vi "UART Config Pane.vi"(6 "_SubPanelMessages":refnum<notifier>, 9 "_myEmbeddedToFrameEvent":T5, 10 "_myEmbedded.Exit":refnum<user-event>, 11 "_Property Bundle":cluster{"Name":string, "Value":variant}[](array[cluster])) -> (1 "_Connection Informations":T1, 2 "_Scripter Input":T7)   [LabVIEW 2021]
doc: "Writes data to or reads data from a Universal Asynchronous Receiver/Transmitter (UART) device."
uses:
  <vilib>/myRIO/Common/Express VI Framework/xctls/myRIO Channel Name/myRIO Channel Name.xctl
  <vilib>/myRIO/Common/Express VI Framework/typedefs/Config Pane to Framework Ref.ctl
  <vilib>/myRIO/Common/Express VI Framework/typedefs/Data Validate Ref.ctl
  <vilib>/myRIO/Common/Express VI Framework/typedefs/Scripter Input.ctl
  <vilib>/myRIO/Common/Express VI Framework/typedefs/WireThrough Terminal Names.ctl
  <vilib>/myRIO/Common/Express VI Framework/typedefs/Instrument Driver Method Descriptor Array.ctl
  <vilib>/myRIO/Common/Express VI Framework/typedefs/Instrument Driver Method Descriptor.ctl
  <vilib>/myRIO/Common/Express VI Framework/typedefs/Sub Panel Messages.ctl
  <vilib>/myRIO/Common/Express VI Framework/typedefs/Connection Informations.ctl
  <vilib>/myRIO/Common/Instrument Driver Framework/Utilities/typedefs/Channel Types.ctl
  <vilib>/myRIO/Instrument Drivers/Onboard IO/UART/typedef/VISA Configuration.ctl
  <vilib>/myRIO/Instrument Drivers/Onboard IO/UART/UART.lvlib
panel:
  in  "Read all Available?":bool
  in  "Mode":enum32{"Write", "Read"}(radio) caption="Mode:"
  in  "Baud rate:":u32(ring)=9600 items=["110"=110, "300"=300, "600"=600, "1,200"=1200, "2,400"=2400, "4,800"=4800, "9,600"=9600, "19,200"=19200, "38,400"=38400, "57,600"=57600, "115,200"=115200, "230,400"=230400]
  in  "Stop bits:":u16(ring)=10 items=["1.0"=10, "2.0"=20]
  in  "Parity:":u16(ring) items=["Even"=2, "Odd"=1, "None"=0]
  in  "Data bits:":u16(ring)=8 items=["7"=7, "8"=8]
  out "_Channel Details:":string caption="Connections:"
  in  "Channel:":u16(xcontrol)
  in  "_Default Alias String":string
  in  "_VI Default Name (Edit and make value default)":string="UART"
  in  "Name:":string caption="Node name:"
  in  "_WireThrough Info (Edit and make value default)":T2={"WireThrough Top In"="VISA resource name in", "WireThrough Bottom In"="error in (no error)", "WireThrough Top Out"="VISA resource name out", "WireThrough Bottom Out"="error out"}
  in  "_Template Array (Edit and make value default)":T3=[{"Function Name"="Open", "VI Path"=path "<vilib>/myRIO/Instrument Drivers/Onboard IO/UART/vis", "Script"=FALSE, "Inputs"=[{"name"="VISA resource name in", "value"=variant, "Config Pane Only"=TRUE, "Build Array"=FALSE, "Bundle Cluster"=FALSE, "Show Term"=FALSE, "alias"=[], "Required Input"=FALSE}], "Outputs"=[], "VI Class"=enum."Open", "Controls Refs[]"=[], "Inline"=FALSE}, {"Function Name"="Configure", "VI Path"=path "<vilib>/myRIO/Instrument Drivers/Onboard IO/UART/vis", "Script"=TRUE, "Inputs"=[{"name"="VISA resource name in", "value"=variant, "Config Pane Only"=TRUE, "Build Array"=FALSE, "Bundle Cluster"=FALSE, "Show Term"=FALSE, "alias"=[], "Required Input"=FALSE}, {"name"="VISA Configuration", "value"=variant, "Config Pane Only"=TRUE, "Build Array"=FALSE, "Bundle Cluster"=FALSE, "Show Term"=FALSE, "alias"=[], "Required Input"=FALSE}], "Outputs"=[], "VI Class"=enum."Configure", "Controls Refs[]"=[], "Inline"=TRUE}, {"Function Name"="Write", "VI Path"=path "<vilib>/myRIO/Instrument Drivers/Onboard IO/UART/vis", "Script"=FALSE, "Inputs"=[{"name"="Characters to Write", "value"=variant, "Config Pane Only"=FALSE, "Build Array"=FALSE, "Bundle Cluster"=FALSE, "Show Term"=TRUE, "alias"=[], "Required Input"=TRUE}], "Outputs"=[{"name"="Character Count", "value"=variant, "Show Term"=TRUE, "Index Array"=FALSE, "Unbundle Cluster"=FALSE, "alias"=[]}], "VI Class"=enum."Data", "Controls Refs[]"=[], "Inline"=TRUE}, {"Function Name"="Read", "VI Path"=path "<vilib>/myRIO/Instrument Drivers/Onboard IO/UART/vis", "Script"=FALSE, "Inputs"=[{"name"="Character Count", "value"=variant, "Config Pane Only"=FALSE, "Build Array"=FALSE, "Bundle Cluster"=FALSE, "Show Term"=TRUE, "alias"=[], "Required Input"=FALSE}], "Outputs"=[{"name"="Characters Read", "value"=variant, "Show Term"=TRUE, "Index Array"=FALSE, "Unbundle Cluster"=FALSE, "alias"=[]}], "VI Class"=enum."Data", "Controls Refs[]"=[], "Inline"=TRUE}, {"Function Name"="Read All", "VI Path"=path "<vilib>/myRIO/Instrument Drivers/Onboard IO/UART/vis", "Script"=FALSE, "Inputs"=[], "Outputs"=[{"name"="Characters Read", "value"=variant, "Show Term"=TRUE, "Index Array"=FALSE, "Unbundle Cluster"=FALSE, "alias"=[]}], "VI Class"=enum."Data", "Controls Refs[]"=[], "Inline"=TRUE}, {"Function Name"="Close", "VI Path"=path "<vilib>/myRIO/Instrument Drivers/Onboard IO/UART/vis", "Script"=FALSE, "Inputs"=[], "Outputs"=[], "VI Class"=enum."Close", "Controls Refs[]"=[], "Inline"=TRUE}, {"Function Name"="Close UART", "VI Path"=path "<vilib>/myRIO/Instrument Drivers/Onboard IO/UART/vis", "Script"=FALSE, "Inputs"=[], "Outputs"=[], "VI Class"=enum."Close", "Controls Refs[]"=[], "Inline"=TRUE}]
  in  "_Test Close":bool
  # "User Visible Area"
  # "NOTE: Tab Order has been set\nfor this Front Panel.\n\nSee Edit>>Set Tabbing Order...\n\nAll controls that are not visible at \nruntime are excluded from Tabbing order\n\nTo exlude a control from context\nhelp prefix its label text with a '-'"
  # "Communication settings"
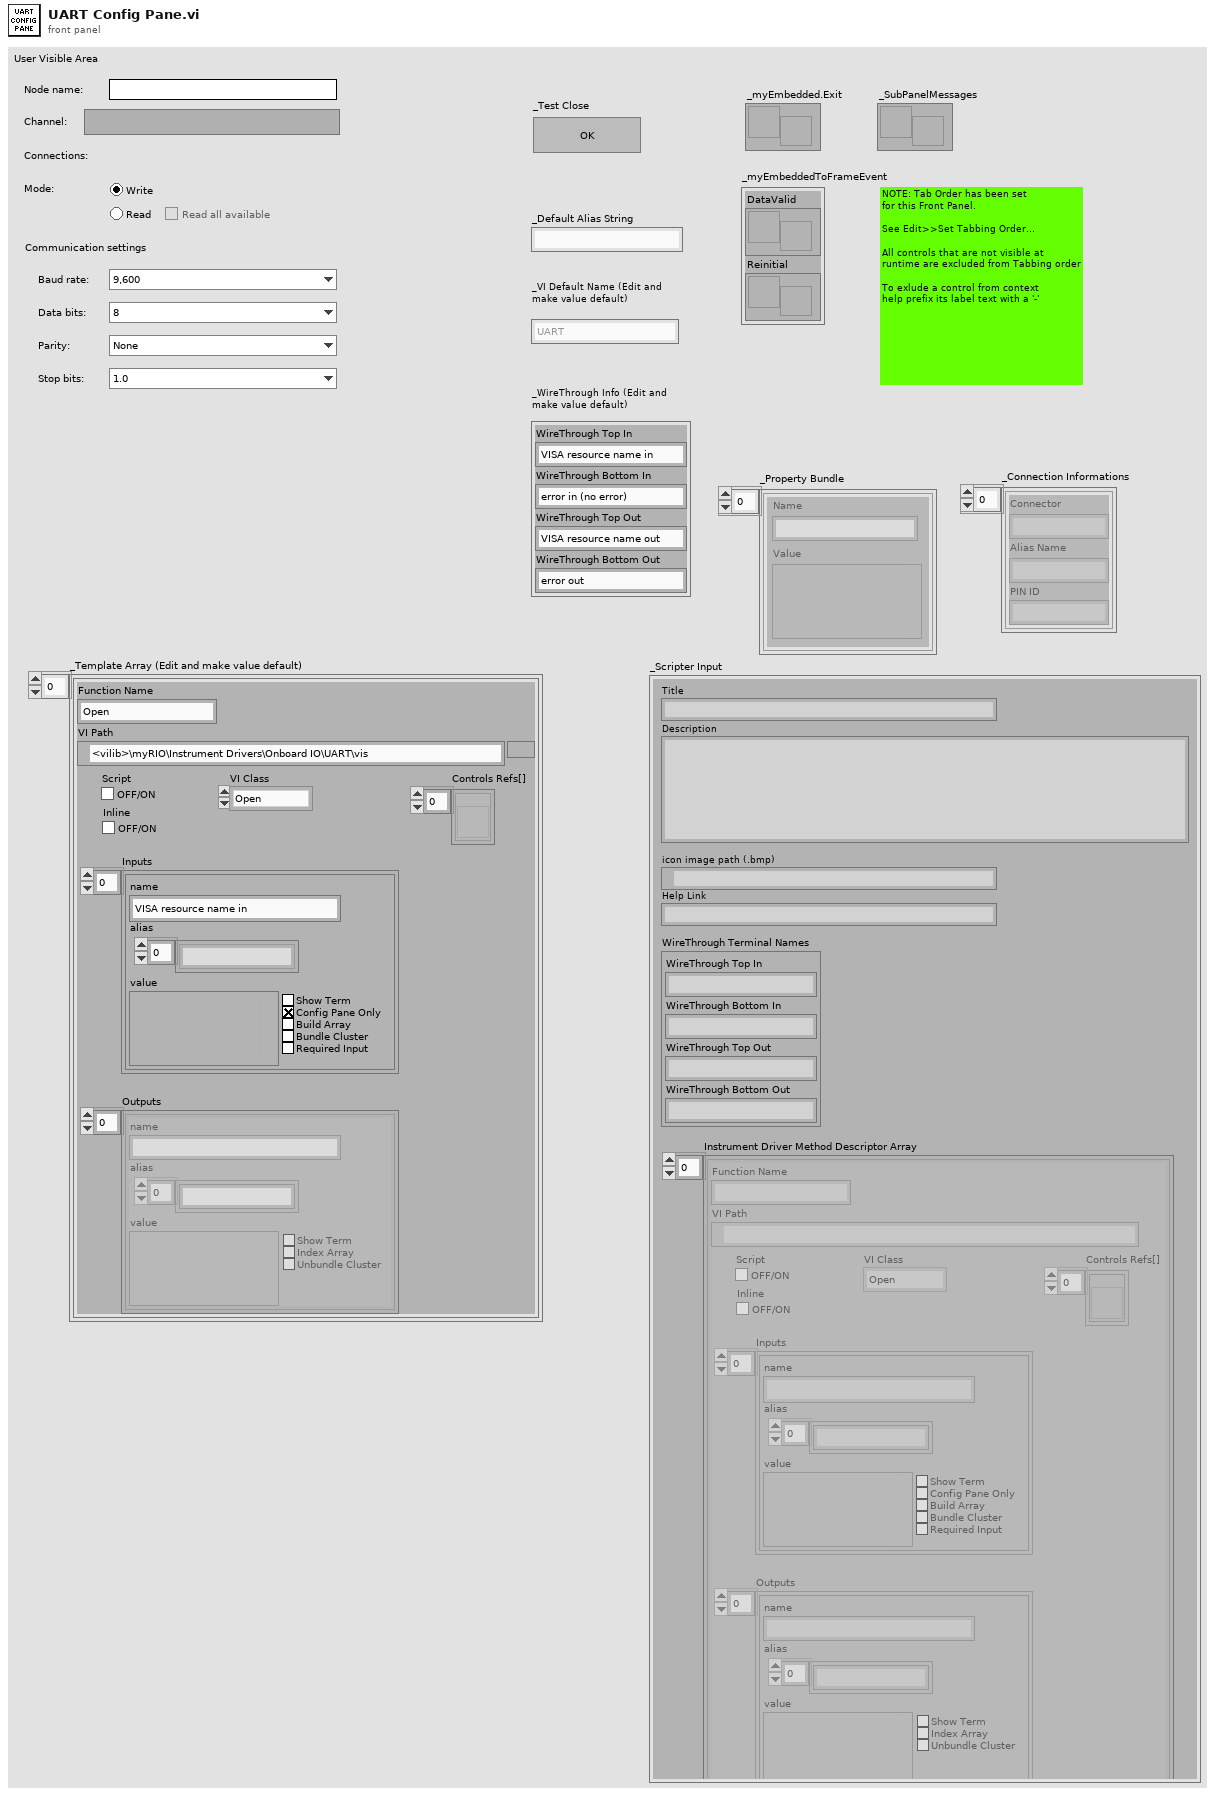
[diagram p1: front panel]
types:
  T1 = typedef "Connection Informations.ctl" = cluster{"Connector":string, "Alias Name":string, "PIN ID":string}[]
  T2 = typedef "WireThrough Terminal Names.ctl" = cluster{"WireThrough Top In":string, "WireThrough Bottom In":string, "WireThrough Top Out":string, "WireThrough Bottom Out":string}
  T3 = typedef "Instrument Driver Method Descriptor Array.ctl" = T4[]
  T4 = typedef "Instrument Driver Method Descriptor.ctl" = cluster{"Function Name":string, "VI Path":path, "Script":bool, "Inputs":cluster{"name":string, "value":variant, "Config Pane Only":bool, "Build Array":bool, "Bundle Cluster":bool, "Show Term":bool, "alias":string[], "Required Input":bool}[], "Outputs":cluster{"name":string, "value":variant, "Show Term":bool, "Index Array":bool, "Unbundle Cluster":bool, "alias":string[]}[], "VI Class":enum16{"Open", "Configure", "Data", "Manage", "Close"}, "Controls Refs[]":refnum<vi>[], "Inline":bool}
  T5 = typedef "Config Pane to Framework Ref.ctl" = cluster{"DataValid":T6, "Reinitial":refnum<user-event>}
  T6 = typedef "Data Validate Ref.ctl" = refnum<user-event>
  T7 = typedef "Scripter Input.ctl" = cluster{"Title":string, "Description":string, "icon image path (.bmp)":path, "Help Link":string, "WireThrough Terminal Names":T2, "Instrument Driver Method Descriptor Array":T3}
  T8 = enum8{"Enabled", "Disabled", "Disabled and Grayed Out"}
  T9 = typedef "Channel Types.ctl" = enum32{"Unknown", "AI", "AO", "DIO - DI", "DIO", "DIO - DO", "I2C", "PWM", "Encoder", "SPI", "UART", "Accelerometer", "DIO - LED", "DIO - Button", "AI (N Samples)", "AudioIn (N Samples)", "AO (N Samples)", "AudioOut (N Samples)", "DI (N Samples)", "DO (N Samples)", "AI IRQ", "DI IRQ", "Timer IRQ", "RSL", "Relay", "CAN", "AI (Continuous)", "AO (Continuous)"}
  T10 = typedef "Channel Info.ctl" = cluster{"Channel Name":string, "Alias":string, "Used?":bool, "Not Support?":bool, "Property Bundle":cluster{"Name":string, "Value":variant}[]}
  T11 = typedef "LVStringsAndValuesArrayTypeDef_U32.ctl" = cluster{"String":string, "Value":u32}[]
  T12 = typedef "Sub Panel Messages.ctl" = enum16{"Initialized"}
  T13 = cluster{"Connector":string, "Alias Name":string, "PIN ID":string}
  T14 = typedef "UART.lvlib/VISA Configuration.ctl" = cluster{"baud rate (9600)":u32, "data bits (8)":u16, "parity (0:none)":enum16{"None", "Odd", "Even", "Mark", "Space"}, "stop bits (10: 1 bit)":u16, "flow control (0:none)":u16, "termination char\n(0xA = '\\n' = LF) ":u8, "Enable Termination\nChar (T)":bool, "timeout (10sec)":u32}
  T15 = cluster{"name":string, "value":variant, "Config Pane Only":bool, "Build Array":bool, "Bundle Cluster":bool, "Show Term":bool, "alias":string[], "Required Input":bool}[]
  T16 = cluster{"name":string, "value":variant, "Config Pane Only":bool, "Build Array":bool, "Bundle Cluster":bool, "Show Term":bool, "alias":string[], "Required Input":bool}
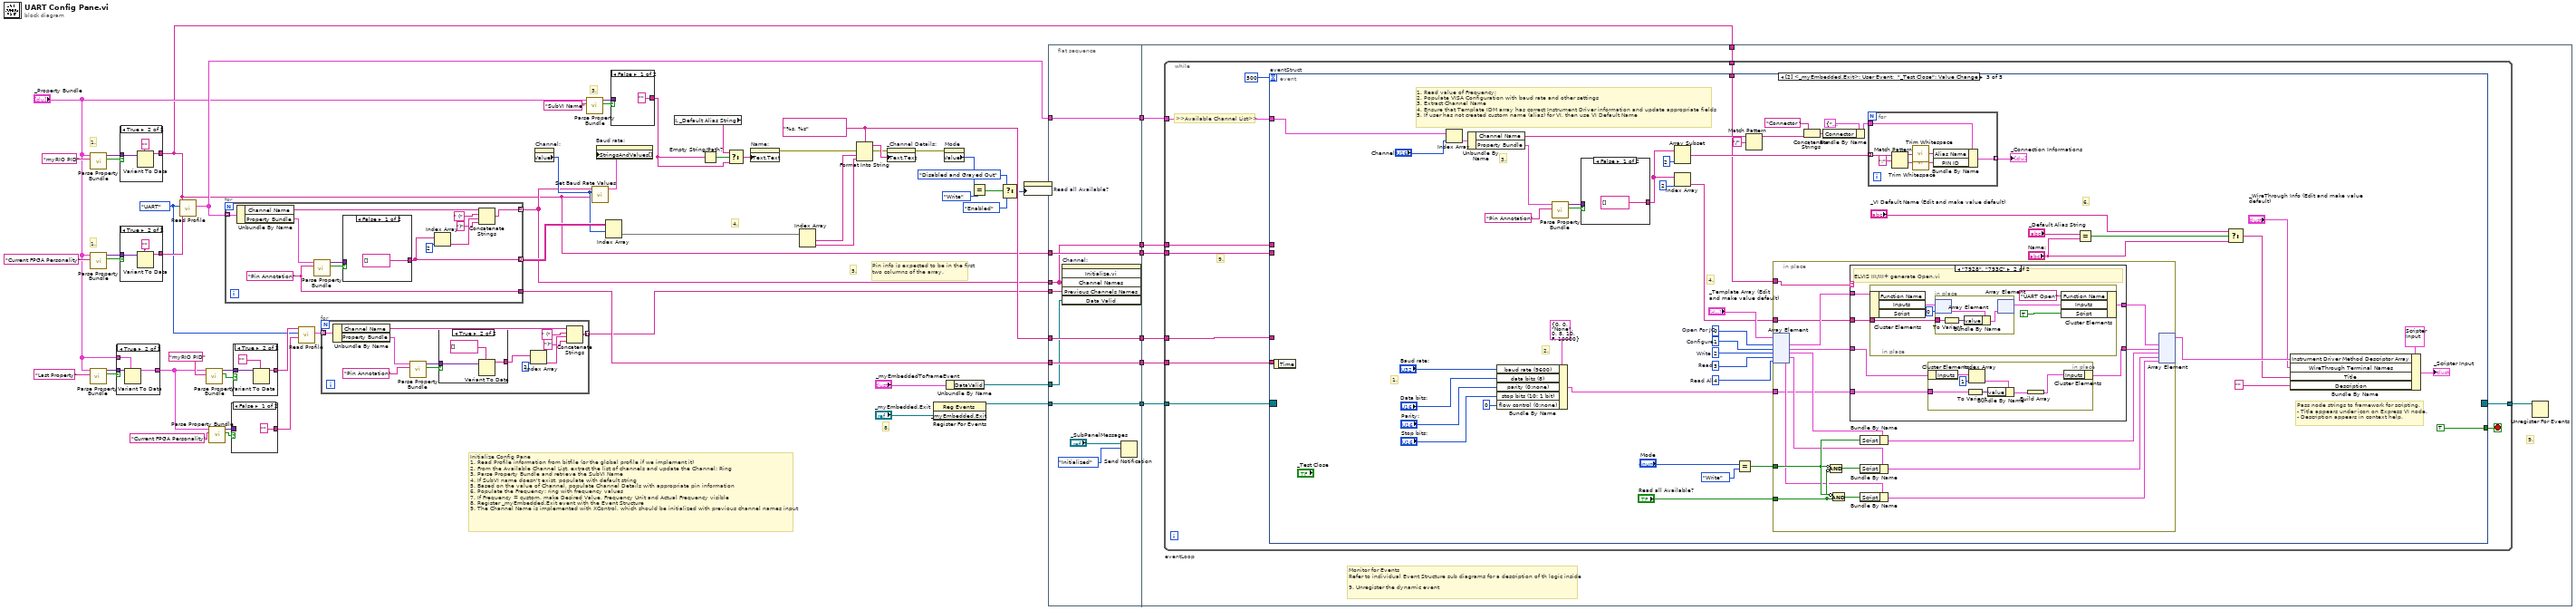
[diagram p0: block diagram]
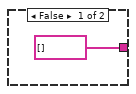
[diagram p2: hidden frame]
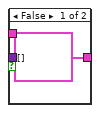
[diagram p3: hidden frame]
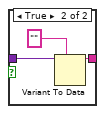
[diagram p4: hidden frame]
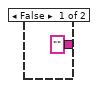
[diagram p5: hidden frame]
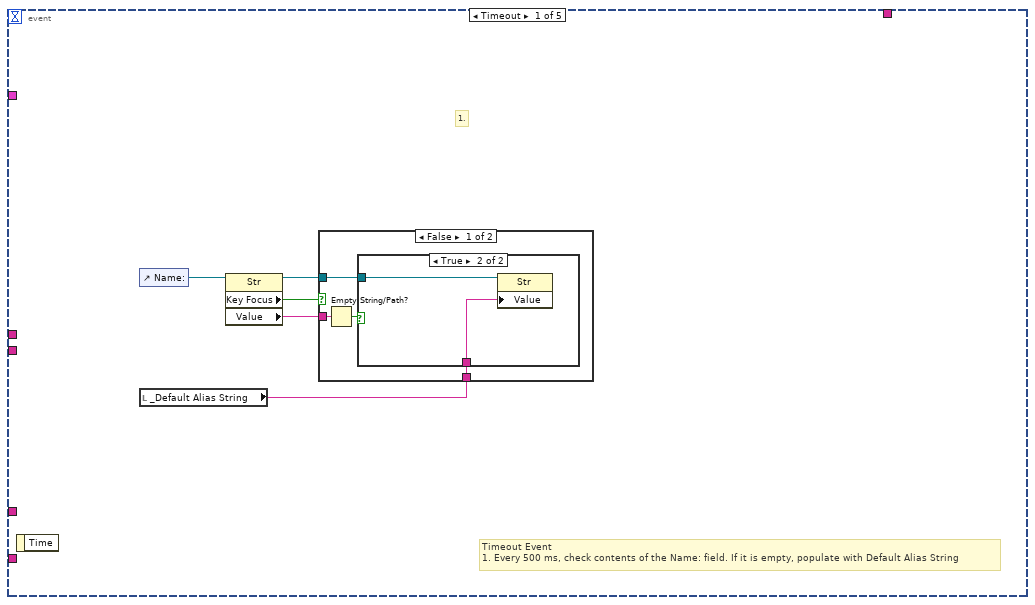
[diagram p6: hidden frame]
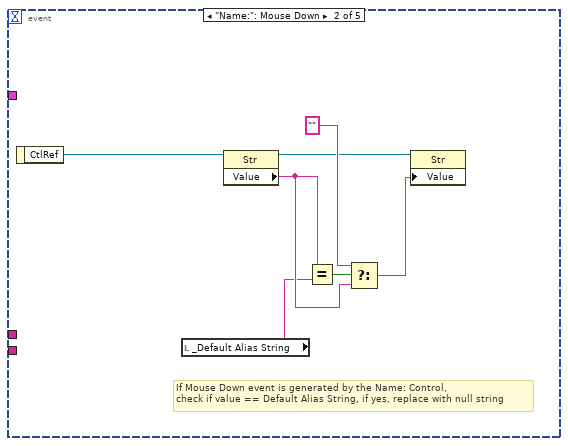
[diagram p9: hidden frame]
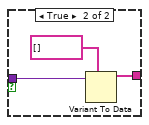
[diagram p10: hidden frame]
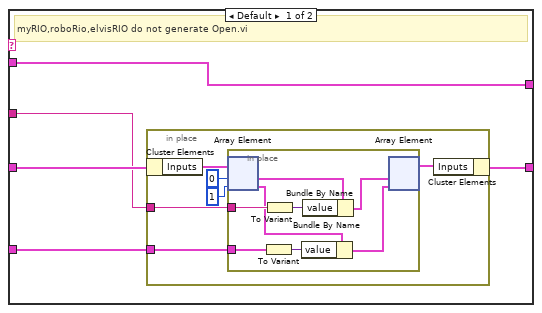
[diagram p11: hidden frame]
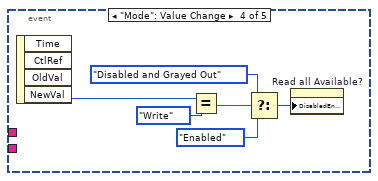
[diagram p12: hidden frame]
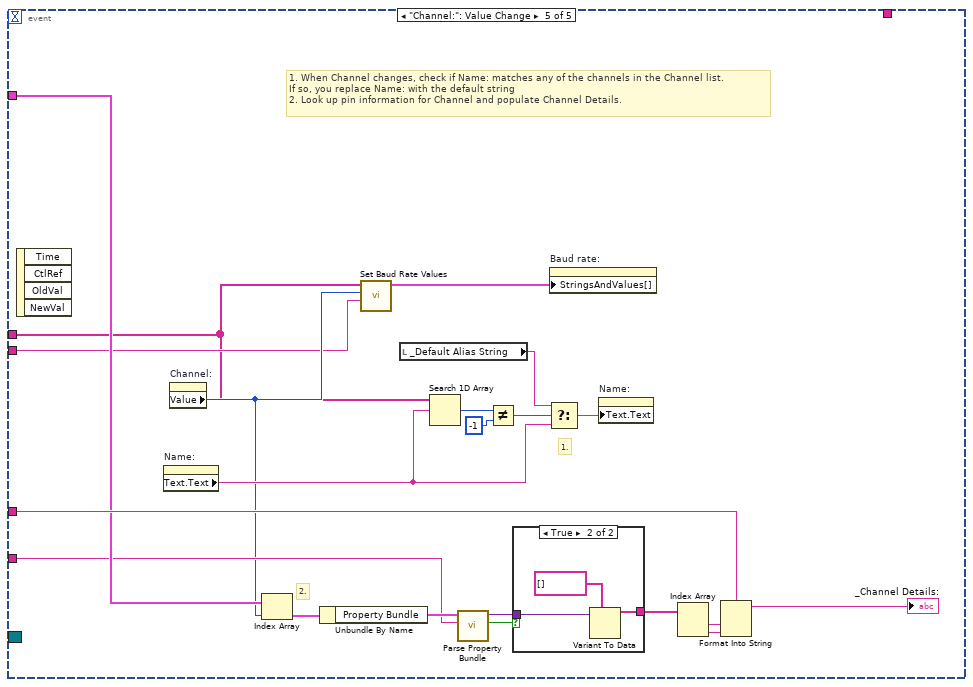
[diagram p13: hidden frame]
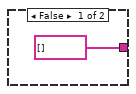
[diagram p14: hidden frame]
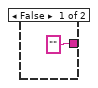
[diagram p15: hidden frame]
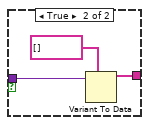
[diagram p16: hidden frame]
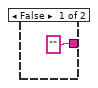
[diagram p17: hidden frame]
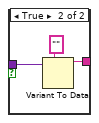
[diagram p18: hidden frame]
diagram:
  w9 = Channel_Types."UART" ("Channel to Read")
  w50 = "%s, %s"
  # "1."
  # "Pin info is expected to be in the first two columns of the array."
  # "1."
  # "8."
  # "5."
  # "4."
  # "3."
  # "Initialize Config Pane\n1. Read Profile information from bitfile (or the global profile if we implement it)\n2. From the Available Channel List, extract the list of channels and update the Channel: Ring\n3. Parse Property Bundle and retrieve the SubVI Name\n4. If SubVI name doesn't exist, populate with default string\n5. Based on the value of Channel, populate Channel Details with appropriate pin information\n6. Populate the Frequency: ring with frequency values\n7. If Frequency = custom, make Desired Value, Frequency Unit and Actual Frequency visible\n8. Register _myEmbedded.Exit event with the Event Structure \n9. The Channel Name is implemented with XControl, which should be initialized with previous channel names input"
  n1 = call <vilib>:"Parse Property Bundle.vi"("Name"="Last Property", "Property Bundle"="_Property Bundle") -> ("Found?"=w12:bool, "Value"=w13:variant)  [unwired: 8 in]
  n2 = call <vilib>:"Parse Property Bundle.vi"("Name"="myRIO PID", "Property Bundle"="_Property Bundle") -> ("Found?"=w45:bool, "Value"=w46:variant)  [unwired: 8 in]
  n3 = call <vilib>:"Parse Property Bundle.vi"("Name"="Current FPGA Personality", "Property Bundle"="_Property Bundle") -> ("Found?"=w32:bool, "Value"=w31:variant)  [unwired: 8 in]
  n4 = case shown="True" w12 {
    tunnel: w13 -> [_ w65]
    tunnel: [cluster{"Name":string, "Value":variant}[] [] ("_Property Bundle") w64] -> w11
    tunnel: "_Property Bundle" -> [_ w63]
    frame False {
    }
    frame True {
      n5 = Variant To Data(type=w63, Variant=w65) -> (data=w64:cluster{"Name":string, "Value":variant}[])  [unwired: 1 in, 1 out]
    }
  }
  n6 = case shown="True" w45 {
    tunnel: w46 -> [_ w69]
    tunnel: ["" ("Name") w67] -> w1
    frame False {
    }
    frame True {
      n7 = Variant To Data(type="" ("Name"), Variant=w69) -> (data=w67:string)  [unwired: 1 in, 1 out]
    }
  }
  n8 = case shown="True" w32 {
    tunnel: w31 -> [_ w73]
    tunnel: ["" ("Name") w71] -> w29
    frame False {
    }
    frame True {
      n9 = Variant To Data(type="" ("Name"), Variant=w73) -> (data=w71:string)  [unwired: 1 in, 1 out]
    }
  }
  n10 = call <vilib>:"Read Profile.vi"("FPGA Name"=w29, "Channel to Read"=w9, "myRIO PID"=w1) -> ("Channel List Out"=w44:T10[])  [unwired: 7 in, 1 out]
  n11 = call <vilib>:"Parse Property Bundle.vi"("Name"="myRIO PID", "Property Bundle"=w11) -> ("Found?"=w21:bool, "Value"=w20:variant)  [unwired: 8 in]
  n12 = call <vilib>:"Parse Property Bundle.vi"("Name"="Current FPGA Personality", "Property Bundle"=w11) -> ("Found?"=w16:bool, "Value"=w17:variant)  [unwired: 8 in]
  n13 = for {
    tunnel: [w83] -> w3 mode=indexing
    tunnel: w44 -> [w85] mode=indexing
    tunnel: [w79] -> w41 mode=indexing
    tunnel: [w80] -> w42
    w80 = "Pin Annotation" ("Name")
    n14 = Unbundle By Name(w85) -> ("Channel Name"=w84:string, "Property Bundle"=w77:cluster{"Name":string, "Value":variant}[])
    n15 = call <vilib>:"Parse Property Bundle.vi"("Name"=w80, "Property Bundle"=w77) -> ("Found?"=w81:bool, "Value"=w82:variant)  [unwired: 8 in]
    n16 = case shown="False" w81 {
      tunnel: w82 -> [_ w89]
      tunnel: [string[] [] w88] -> w79
      frame False {
      }
      frame True {
        n17 = Variant To Data(type=string[] [], Variant=w89) -> (data=w88:string[])  [unwired: 1 in, 1 out]
      }
    }
    n18 = Index Array(array=w79, index=2) -> (element=w76:string)
    n19 = Concatenate Strings(w84, " (" ("string"), w76, ")" ("string")) -> (w83:string)
  }
  n20 = case shown="False" w16 {
    tunnel: w17 -> [_ w93]
    tunnel: ["" ("Name") w91] -> w15
    frame False {
    }
    frame True {
      n21 = Variant To Data(type="" ("Name"), Variant=w93) -> (data=w91:string)  [unwired: 1 in, 1 out]
    }
  }
  n22 = case shown="True" w21 {
    tunnel: w20 -> [_ w97]
    tunnel: ["" ("Name") w95] -> w22
    frame False {
    }
    frame True {
      n23 = Variant To Data(type="" ("Name"), Variant=w97) -> (data=w95:string)  [unwired: 1 in, 1 out]
    }
  }
  n24 = call <vilib>:"Read Profile.vi"("FPGA Name"=w15, "Channel to Read"=w9, "myRIO PID"=w22) -> ("Channel List Out"=w8:T10[])  [unwired: 7 in, 1 out]
  n25 = for {
    tunnel: [w107] -> w2 mode=indexing
    tunnel: w8 -> [w109] mode=indexing
    n26 = Unbundle By Name(w109) -> ("Channel Name"=w108:string, "Property Bundle"=w101:cluster{"Name":string, "Value":variant}[])
    n27 = call <vilib>:"Parse Property Bundle.vi"("Name"="Pin Annotation", "Property Bundle"=w101) -> ("Found?"=w105:bool, "Value"=w106:variant)  [unwired: 8 in]
    n28 = case shown="True" w105 {
      tunnel: w106 -> [_ w113]
      tunnel: [string[] [] w112] -> w103
      frame False {
      }
      frame True {
        n29 = Variant To Data(type=string[] [], Variant=w113) -> (data=w112:string[])  [unwired: 1 in, 1 out]
      }
    }
    n30 = Index Array(array=w103, index=2) -> (element=w100:string)
    n31 = Concatenate Strings(w108, " (" ("string"), w100, ")" ("string")) -> (w107:string)
  }
  n32 = property on="Channel:" class="myRIO Channel Name (strict)"() -> ("Value"=w4:u16)  [unwired: 2 in, 2 out]
  n33 = call <vilib>:"Parse Property Bundle.vi"("Name"="SubVI Name", "Property Bundle"="_Property Bundle") -> ("Found?"=w56:bool, "Value"=w55:variant)  [unwired: 8 in]
  n34 = call <vilib>:"Set Baud Rate Values.vi"("PID"=w1, "Channel Index"=w4, "Channel Str"=w3) -> ("Baud Rate Strings And Values"=w24:T11)  [unwired: 8 in]
  n35 = property on="Baud rate:" class="Ring (strict)"("StringsAndValues[]"=w24) -> ()  [unwired: 2 in, 2 out]
  n36 = Index Array(array=w41, index (row)=w4) -> (element=w40:string[])  [unwired: 1 in]
  n37 = case shown="False" w56 {
    tunnel: w55 -> [_ w117]
    tunnel: ["" ("Name") w115] -> w54
    frame False {
    }
    frame True {
      n38 = Variant To Data(type="" ("Name"), Variant=w117) -> (data=w115:string)  [unwired: 1 in, 1 out]
    }
  }
  n39 = local read "_Default Alias String"() -> (w58:string)
  n40 = Empty String/Path?(string/path=w54) -> (empty?=w59:bool)
  n41 = Select(t=w58, s=w59, f=w54) -> (s? t:f=w43:string)
  n42 = property on="Name:" class="Str"("Text.Text"=w43) -> (error out=w53:errorcluster)  [unwired: 2 in, 1 out]
  n43 = Index Array(array=w40) -> (element #1=w49:string, element #2=w48:string)  [unwired: 2 in]
  n44 = Format Into String(format string=w50, error in=w53, w49, w48) -> (resulting string=w52:string, error out=w51:errorcluster)  [unwired: 1 in]
  n45 = property on="_Channel Details:" class="Str"(error in=w51, "Text.Text"=w52) -> (error out=w34:errorcluster)  [unwired: 1 in, 1 out]
  n46 = register-events("_myEmbedded.Exit") -> (reference out=w61:refnum<event-registration>)  [unwired: 2 in, 1 out]
  n47 = property on="Mode" class="RadioBtnsControl (strict)"(error in=w34) -> ("Value"=w33:enum32{"Write", "Read"})  [unwired: 1 in, 2 out]
  n48 = Unbundle By Name("_myEmbeddedToFrameEvent") -> ("DataValid"=w6:T6)
  n49 = Equal?(x=w33, y=enum32{"Write", "Read"}."Write") -> (x = y?=w36:bool)
  n50 = Select(t=T8."Disabled and Grayed Out", s=w36, f=T8."Enabled" ("Disabled")) -> (s? t:f=w39:T8)
  n51 = property on="Read all Available?" class="Bool (strict)"("DisabledEnum"=w39) -> ()  [unwired: 2 in, 2 out]
  n52 = flat-sequence {
    tunnel: w42 -> [w124]
    tunnel: w44 -> [w125]
    tunnel: w50 -> [w126]
    tunnel: w61 -> [w127]
    tunnel: [w127] -> w28
    tunnel: [w126] -> w27
    tunnel: [w125] -> w26
    tunnel: [w124] -> w25
    tunnel: [w121] -> w23
    tunnel: w1 -> [w121]
    tunnel: w6 -> [w118]
    tunnel: w2 -> [w119]
    tunnel: w3 -> [w120]
    tunnel: [w120] -> w5
    tunnel: w28 -> [w135]
    tunnel: w27 -> [w133]
    tunnel: w26 -> [w132]
    tunnel: w25 -> [w131]
    tunnel: w23 -> [w130]
    tunnel: w5 -> [w129]
    tunnel: w1 -> [w128]
    frame #0 {
      n53 = invoke on="Channel:" class="myRIO Channel Name (strict)" method="Initialize.vi"("Channel Names"=w120, "Previous Channels Names"=w119, "Data Valid"=w118) -> ()  [unwired: 3 in, 6 out]
      n54 = Send Notification(notification=Sub_Panel_Messages."Initialized", notifier="_SubPanelMessages") -> ()  [unwired: 1 in, 2 out]
    }
    frame #1 {
      # "9."
      # "Monitor for Events\nRefer to individual Event Structure sub diagrams for a description of th logic inside\n\n9. Unregister the dynamic event"
      n55 = while "eventLoop" {
        tunnel: w135 -> [w144]
        tunnel: [w143] -> w134
        tunnel: w132 -> [w141]
        tunnel: w133 -> [w140]
        tunnel: w131 -> [w139]
        tunnel: w130 -> [w138]
        tunnel: w129 -> [w137]
        tunnel: w128 -> [w136]
        stop <- w145 stop-if-true
        # "9."
        # ">>Available Channel List>>"
        n56 = event "eventStruct" shown="[2] <_myEmbedded.Exit>: User Event;  \"_Test Close\": Value Change" {
          selector: w144 -> [_ _ _ _ _]
          dyn-events: [_ _ _ _ _] -> w143
          timeout: 500 -> [_ _ _ _ _]
          tunnel: [_ _ TRUE ("_Test Close") _ _] -> w145
          tunnel: w141 -> [_ _ w211 _ w296]
          tunnel: w140 -> [_ _ _ _ w303]
          tunnel: w139 -> [_ _ _ _ w295]
          tunnel: w138 -> [_ _ _ _ w291]
          tunnel: w137 -> [_ _ _ _ w290]
          tunnel: w136 -> [_ _ w166 _ _]
          event Timeout {
            # "Timeout Event\n1. Every 500 ms, check contents of the Name: field. If it is empty, populate with Default Alias String"
            # "1."
            n57 = event-data() -> ()  [unwired: 1 in, 1 out]
            n58 = control-ref of="Name:"() -> (w148:refnum<vi>)
            n59 = local read "_Default Alias String"() -> (w146:string)
            n60 = property on="Property Node" class="Str"(reference=w148) -> (reference out=w147:refnum<vi>, "Key Focus"=w149:bool, "Value"=w150:string)  [unwired: 1 in, 1 out]
            n61 = case shown="False" w149 {
              tunnel: w150 -> [w154 _]
              tunnel: w147 -> [w152 _]
              tunnel: w146 -> [w151 _]
              frame False {
                n62 = Empty String/Path?(string/path=w154) -> (empty?=w153:bool)
                n63 = case shown="True" w153 {
                  tunnel: w152 -> [_ w156]
                  tunnel: w151 -> [_ w155]
                  frame False {
                  }
                  frame True {
                    n64 = property on="Property Node" class="Str"(reference=w156, "Value"=w155) -> ()  [unwired: 1 in, 2 out]
                  }
                }
              }
              frame True {
              }
            }
          }
          event "Name:": Mouse Down {
            # "If Mouse Down event is generated by the Name: Control,\ncheck if value == Default Alias String, if yes, replace with null string"
            n65 = event-data() -> ("CtlRef"=w163:refnum<vi>)  [unwired: 1 in]
            n66 = local read "_Default Alias String"() -> (w157:string)
            n67 = property class="Str"(reference=w163) -> (reference out=w159:refnum<vi>, "Value"=w158:string)  [unwired: 1 in, 1 out]
            n68 = Equal?(x=w158, y=w157) -> (x = y?=w162:bool)
            n69 = Select(t="", s=w162, f=w158) -> (s? t:f=w160:string)
            n70 = property class="Str"(reference=w159, "Value"=w160) -> ()  [unwired: 1 in, 2 out]
          }
          event User Event; "_Test Close": Value Change {
            w167 = 0  # Open For JC
            w179 = 4  # Read All
            w190 = 3  # Read
            w210 = 2  # Write
            w207 = 1  # Configure
            # "3."
            # "2."
            # "1. Read value of Frequency:\n2. Populate VISA Configuration with baud rate and other settings\n3. Extract Channel Name\n4. Ensure that Template IDM array has correct Instrument Driver information and update appropriate fields\n5. If user has not created custom name (alias) for VI, then use VI Default Name"
            # "6."
            # "4."
            # "1."
            # "Pass node strings to framework for scripting.\n- Title appears under icon on Express VI node.\n- Description appears in context help."
            n71 = event-data() -> ()  [unwired: 1 in, 1 out]
            n72 = Index Array(array=w211, index="Channel:") -> (element=w188:T10)
            n73 = Unbundle By Name(w188) -> ("Channel Name"=w169:string, "Property Bundle"=w183:cluster{"Name":string, "Value":variant}[])
            n74 = Bundle By Name(cluster=T14 {"baud rate (9600)"=0, "data bits (8)"=0, "parity (0:none)"=enum."None", "stop bits (10: 1 bit)"=0, "flow control (0:none)"=8, "termination char\n(0xA = '\\n' = LF) "=10, "Enable Termination\nChar (T)"=FALSE, "timeout (10sec)"=10000} ("VISA Configuration"), "baud rate (9600)"="Baud rate:", "data bits (8)"="Data bits:", "parity (0:none)"="Parity:", "stop bits (10: 1 bit)"="Stop bits:", "flow control (0:none)"=u16 0) -> (w164:T14)
            n75 = call <vilib>:"Parse Property Bundle.vi"("Name"="Pin Annotation", "Property Bundle"=w183) -> ("Found?"=w186:bool, "Value"=w187:variant)  [unwired: 8 in]
            n76 = case shown="False" w186 {
              tunnel: w187 -> [_ w224]
              tunnel: [string[] [] w223] -> w172
              frame False {
              }
              frame True {
                n77 = Variant To Data(type=string[] [], Variant=w224) -> (data=w223:string[])  [unwired: 1 in, 1 out]
              }
            }
            n78 = Array Subset(array=w172, length=2) -> (w170:string[])  [unwired: 1 in]
            n79 = Index Array(array=w172, index=2) -> (element=w165:string)
            n80 = Equal?(x="Mode", y=enum32{"Write", "Read"}."Write") -> (x = y?=w181:bool)
            n81 = Match Pattern(string=w169, regular expression="/") -> (before substring=w176:string)  [unwired: 1 in, 3 out]
            n82 = in-place {
              in-place-border: w181 -> [w241]
              in-place-border: "Read all Available?" -> [w236]
              in-place-border: w166 -> [w231]
              in-place-border: w165 -> [w227]
              in-place-border: w164 -> [w226]
              n83 = in-place-array #1("_Template Array (Edit and make value default)", w167, w207, w210, w190, w179) -> (w230:T4, w225:T4, w240:T4, w239:T4, w235:T4)
              n84 = Compound Arithmetic op=AND(invert w241, invert w236) -> (w233:bool)
              n85 = Compound Arithmetic op=AND(invert w241, w236) -> (w232:bool)
              n86 = case shown="\"7928\", \"793C\"" w231 {
                tunnel: w230 -> [w246 w265]
                tunnel: [w246 w263] -> w229
                tunnel: [w243 w266] -> w228
                tunnel: w227 -> [w242 w264]
                tunnel: w226 -> [w245 w261]
                tunnel: w225 -> [w244 w262]
                frame Default {
                  # "myRIO,roboRio,elvisRIO do not generate Open.vi"
                  n87 = in-place {
                    in-place-border: w242 -> [w251]
                    in-place-border: w245 -> [w247]
                    n88 = in-place-cluster #2(w244) -> ("Inputs"=w252:T15)
                    n89 = in-place {
                      in-place-border: w251 -> [w257]
                      in-place-border: w247 -> [w253]
                      n90 = in-place-array #3(w252, 0, 1) -> (w260:T16, w255:T16)
                      n91 = To Variant(anything=w253) -> (Variant=w256:variant)
                      n92 = To Variant(anything=w257) -> (Variant=w258:variant)
                      n93 = Bundle By Name(cluster=w255, "value"=w256) -> (w254:T16)
                      n94 = Bundle By Name(cluster=w260, "value"=w258) -> (w259:T16)
                      n95 = in-place-array #3(w259, w254) -> (w250:T15)  [unwired: 2 out]
                    }
                    n96 = in-place-cluster #2("Inputs"=w250) -> (w243:T4)
                  }
                }
                frame "7928", "793C" {
                  # "ELVIS III/III+ generate Open.vi"
                  n97 = in-place {
                    in-place-border: w264 -> [w269]
                    n98 = in-place-cluster #4(w265) -> ("Inputs"=w272:T15)  [unwired: 2 out]
                    n99 = in-place {
                      in-place-border: w269 -> [w273]
                      n100 = in-place-array #5(w272, 0) -> (w276:T16)
                      n101 = To Variant(anything=w273) -> (Variant=w274:variant)
                      n102 = Bundle By Name(cluster=w276, "value"=w274) -> (w275:T16)
                      n103 = in-place-array #5(w275) -> (w271:T15)  [unwired: 1 out]
                    }
                    n104 = in-place-cluster #4("Function Name"="UART Open", "Inputs"=w271, "Script"=TRUE) -> (w263:T4)
                  }
                  n105 = in-place {
                    in-place-border: w261 -> [w277]
                    n106 = in-place-cluster #6(w262) -> ("Inputs"=w283:T15)
                    n107 = To Variant(anything=w277) -> (Variant=w281:variant)
                    n108 = Index Array(array=w283, index=1) -> (element=w280:T16)
                    n109 = Bundle By Name(cluster=w280, "value"=w281) -> (w279:T16)
                    n110 = Build Array(w279) -> (w278:T15)
                    n111 = in-place-cluster #6("Inputs"=w278) -> (w266:T4)
                  }
                }
              }
              n112 = Bundle By Name(cluster=w240, "Script"=w241) -> (w238:T4)
              n113 = Bundle By Name(cluster=w239, "Script"=w233) -> (w237:T4)
              n114 = Bundle By Name(cluster=w235, "Script"=w232) -> (w234:T4)
              n115 = in-place-array #1(w229, w228, w238, w237, w234) -> (w209:T3)  [unwired: 5 out]
            }
            n116 = Concatenate Strings("Connector " ("string"), w176) -> (w178:string)
            n117 = Bundle By Name(cluster=T13 {"Connector"="", "Alias Name"="", "PIN ID"=""} ("Connection Information"), "Connector"=w178) -> (w174:T13)
            n118 = for {
              tunnel: w170 -> [w219] mode=indexing
              tunnel: w174 -> [w220]
              tunnel: [w215] -> w168 mode=indexing
              n119 = Match Pattern(string=w219, regular expression=":") -> (before substring=w217:string, after substring=w216:string)  [unwired: 1 in, 2 out]
              n120 = call <vilib>:"Trim Whitespace.vi"("string"=w217) -> ("trimmed string"=w214:string)  [unwired: 1 in]
              n121 = call <vilib>:"Trim Whitespace.vi"("string"=w216) -> ("trimmed string"=w213:string)  [unwired: 1 in]
              n122 = Bundle By Name(cluster=w220, "Alias Name"=w214, "PIN ID"=w213) -> (w215:T13)
            }
            "_Connection Informations" <- w168
            n123 = Equal?(x="_Default Alias String", y="Name:") -> (x = y?=w201:bool)
            n124 = Select(t="_VI Default Name (Edit and make value default)", s=w201, f="Name:") -> (s? t:f=w200:string)
            n125 = Bundle By Name(cluster=T7 {"Title"="", "Description"="", "icon image path (.bmp)"=path "", "Help Link"="", "WireThrough Terminal Names"={"WireThrough Top In"="", "WireThrough Bottom In"="", "WireThrough Top Out"="", "WireThrough Bottom Out"=""}, "Instrument Driver Method Descriptor Array"=[]} ("Scripter Input"), "Instrument Driver Method Descriptor Array"=w209, "WireThrough Terminal Names"="_WireThrough Info (Edit and make value default)", "Title"=w200, "Description"="" ("Title")) -> (→"_Scripter Input":T7)
          }
          event "Mode": Value Change {
            n126 = event-data() -> ("NewVal"=w289:enum32{"Write", "Read"})  [unwired: 1 in, 3 out]
            n127 = Equal?(x=w289, y=enum32{"Write", "Read"}."Write") -> (x = y?=w287:bool)
            n128 = Select(t=T8."Disabled and Grayed Out", s=w287, f=T8."Enabled" ("Disabled")) -> (s? t:f=w284:T8)
            n129 = property on="Read all Available?" class="Bool (strict)"("DisabledEnum"=w284) -> ()  [unwired: 2 in, 2 out]
          }
          event "Channel:": Value Change {
            # "2."
            # "1."
            # "1. When Channel changes, check if Name: matches any of the channels in the Channel list. \nIf so, you replace Name: with the default string\n2. Look up pin information for Channel and populate Channel Details."
            n130 = event-data() -> ()  [unwired: 1 in, 4 out]
            n131 = property on="Name:" class="Str"() -> ("Text.Text"=w307:string)  [unwired: 2 in, 2 out]
            n132 = property on="Channel:" class="myRIO Channel Name (strict)"() -> ("Value"=w293:u16)  [unwired: 2 in, 2 out]
            n133 = Index Array(array=w296, index=w293) -> (element=w298:T10)
            n134 = Unbundle By Name(w298) -> ("Property Bundle"=w297:cluster{"Name":string, "Value":variant}[])
            n135 = call <vilib>:"Set Baud Rate Values.vi"("PID"=w291, "Channel Index"=w293, "Channel Str"=w290) -> ("Baud Rate Strings And Values"=w292:T11)  [unwired: 8 in]
            n136 = local read "_Default Alias String"() -> (w305:string)
            n137 = Search 1D Array(1D array=w290, element=w307) -> (index of element=w310:i32)  [unwired: 1 in]
            n138 = call <vilib>:"Parse Property Bundle.vi"("Name"=w295, "Property Bundle"=w297) -> ("Found?"=w299:bool, "Value"=w300:variant)  [unwired: 8 in]
            n139 = Not Equal?(x=w310, y=-1) -> (x != y?=w308:bool)
            n140 = case shown="True" w299 {
              tunnel: w300 -> [_ w314]
              tunnel: [string[] [] w313] -> w294
              frame False {
              }
              frame True {
                n141 = Variant To Data(type=string[] [], Variant=w314) -> (data=w313:string[])  [unwired: 1 in, 1 out]
              }
            }
            n142 = Select(t=w305, s=w308, f=w307) -> (s? t:f=w306:string)
            n143 = property on="Baud rate:" class="Ring (strict)"("StringsAndValues[]"=w292) -> ()  [unwired: 2 in, 2 out]
            n144 = property on="Name:" class="Str"("Text.Text"=w306) -> ()  [unwired: 2 in, 2 out]
            n145 = Index Array(array=w294) -> (element #1=w302:string, element #2=w301:string)  [unwired: 2 in]
            n146 = Format Into String(format string=w303, w302, w301) -> (resulting string=→"_Channel Details:":string)  [unwired: 2 in, 1 out]
          }
        }
      }
      n147 = Unregister For Events(event registration refnum=w134) -> ()  [unwired: 1 in, 1 out]
    }
  }
